vi "CPP-ZeroChannels.vi"(1 "SecondsToAverage":dbl, 2 "ADAM Ch Names":string[](array[string])=["Tunnel3:StaticP:1", "Tunnel3:StaticP:2", "Tunnel3:StaticP:3", "Tunnel3:StaticP:4", "Tunnel3:StaticP:5", "Tunnel3:StaticP:6", "Tunnel3:StaticP:7", "Tunnel3:StaticP:8"]) -> (0 "Seconds since 1 Jan 1904":dbl)   [LabVIEW 2014]
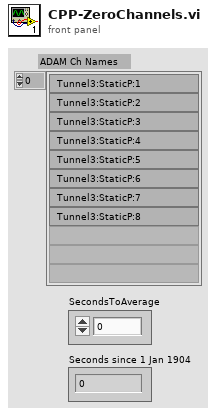
[diagram p1: front panel]
types:
  T1 = typedef "Ch_description_ADAM.ctl" = cluster{"Ch Name":string, "Type":T2, "Function":T3, "Ch State":T4, "Calibration type":T5, "A":dbl, "B":dbl, "C":dbl, "D":dbl, "Comments":string, "Address":T6, "String":string, "Duty":u16}
  T2 = typedef "Module_type_ADAM.ctl" = string
  T3 = typedef "Function_ADAM.ctl" = enum16{"Analogue Input", "Digital Input", "Event counter", "Event rate", "Analogue Output", "Digital Output", "Relay Output"}
  T4 = typedef "Channel_State.ctl" = enum16{"On", "Off", "Always On", "Always Off"}
  T5 = typedef "Calib_type_ADAM.ctl" = enum16{"Raw", "Bx + A", "Cx^2 + Bx + A", "Dx^3 + Cx^2 + Bx + A", "In Band", "Hi-Tec Q", "Hi-Tec M_dot", "Text"}
  T6 = typedef "Address.ctl" = cluster{"Main":i32, "Ch.":i32, "Sub":i32, "Port Name":string}
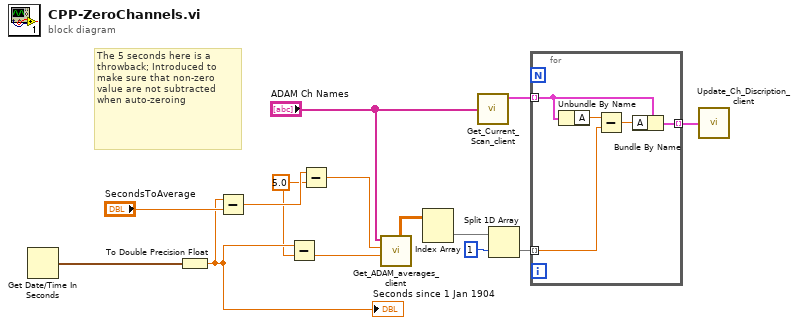
[diagram p0: block diagram]
diagram:
  w1 = 5.0 ("y")
  # "The 5 seconds here is a throwback; Introduced to make sure that non-zero value are not subtracted when auto-zeroing"
  n1 = Get Date/Time In Seconds() -> (seconds since 1Jan1904=w14:timestamp)
  n2 = To Double Precision Float(number=w14) -> (double precision float=w2:dbl)
  "Seconds since 1 Jan 1904" <- w2
  n3 = Subtract(x=w2, y="SecondsToAverage") -> (x-y=w5:dbl)
  n4 = Subtract(x=w2, y=w1) -> (x-y=w3:dbl)
  n5 = Subtract(x=w5, y=w1) -> (x-y=w4:dbl)
  n6 = call "Get_ADAM_averages_client.vi"("End time"=w3, "Start time"=w4, "ADAM Ch Names"="ADAM Ch Names") -> ("DBL values"=w10:dbl[][])  [unwired: 4 in, 4 out]
  n7 = Index Array(array=w10) -> (element=w9:dbl[])  [unwired: 2 in]
  n8 = call "Get_Current_Scan_client.vi"("ADAM Ch Names"="ADAM Ch Names") -> ("Ch Description Array"=w11:T1[])  [unwired: 3 out]
  n9 = Split 1D Array(array=w9, index=1) -> (second subarray=w8:dbl[])  [unwired: 1 out]
  n10 = for {
    tunnel: w11 -> [w17] mode=indexing
    tunnel: w8 -> [w18] mode=indexing
    tunnel: [w15] -> w6 mode=indexing
    n11 = Unbundle By Name(w17) -> ("A"=w19:dbl)
    n12 = Subtract(x=w19, y=w18) -> (x-y=w16:dbl)
    n13 = Bundle By Name(cluster=w17, "A"=w16) -> (w15:T1)
  }
  n14 = call "Update_Ch_Discription_client.vi"("Channels to update In"=w6) -> ()  [unwired: 1 out]
